vi "Set ROI HW lines limit.vi"(8 "error in (no error)":errorcluster) -> (0 "error out":errorcluster)   [LabVIEW 2020]
uses:
  Typedefs/HW config states enum.ctl
  Global Variables/General Globals.vi
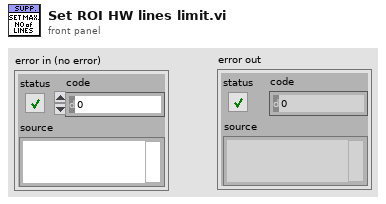
[diagram p1: front panel]
types:
  T1 = typedef "HW config states enum.ctl" = enum16{"Load from file", "Save to file", "Save backup", "Write all", "Read all", "Write XY stage settings", "Write DAQ FPGA settings", "Write Control FPGA settings", "Write Phys Channels", "Write System Config", "Write HW Config", "Save System Config", "Save HW Config", "Clear", "Compare from file"}
  T2 = typedef "Hardware Configuration settings.ctl" = cluster{"Dev. PC":bool, "Swap XY on stage":bool, "No of AOD":u8, "MC Supported":bool, "Axial MC":bool, "Computer MAC address":string, "Externalise Triggers":bool, "Trigger HW config":T3, "DAQmx Chan":T4, "XY stage available":bool, "XY Stage":T5, "Z stage available":bool, "Z Stage config cluster":T6, "Encoder available":bool, "Encoder":T7, "VidRec available":bool, "Cam VidRec":T8, "Laser Power Control HW config":T9, "Laser 1 available":bool, "Laser 1 config cluster":T10, "Prechirper 1 available":bool, "Prechirper 1 config cluster":T11, "Control system.FPGA available?":bool, "Control Sys. HW config":T12, "DAQ FPGA HW Config":T13, "PMT Voltage Range":T17}
  T3 = typedef "Triggers HW config.ctl" = cluster{"Available Device List":i32, "Device Address":string}
  T4 = typedef "DAQmx physical channels cluster.ctl" = cluster{"Pockels AO":tag, "Hard shutter AO":tag, "PMT AOs":tag, "Galvo AOs":tag, "Power meter AI":tag}
  T5 = typedef "XY Stage config cluster.ctl" = cluster{"COM port":refnum<visa-resource-name>, "Baudrate":i32, "Type":string}
  T6 = typedef "Z Stage config cluster.ctl" = cluster{"COM port":refnum<visa-resource-name>, "Baudrate":i32, "Type":string}
  T7 = typedef "Encoder config cluster.ctl" = cluster{"IP address":string, "Port":u16, "Wheel radius (cm)":dbl, "Encoder Trigger":tag}
  T8 = typedef "Cam VidRec HW config setup cluster.ctl" = cluster{"DO flag-Video record":tag, "DO flag-Trial start":tag}
  T9 = typedef "Laser Power Control HW config.ctl" = cluster{"Laser Power Control":string, "Laser Power Modulation Control":enum16{"NI", "FPGA"}}
  T10 = typedef "Laser 1 config cluster.ctl" = cluster{"COM port":refnum<visa-resource-name>, "Baud Rate":i32, "Type":string}
  T11 = typedef "PreChirper 1 config cluster.ctl" = cluster{"Type":string, "Baud Rate":i32, "COM port":refnum<visa-resource-name>}
  T12 = typedef "Control Sys HW config cluster.ctl" = cluster{"Control system.FPGA Type":enum16{"Virtex 5", "Virtex 7"}, "Control system.Network adapter name":string, "Control system.MAC address":string, "Control system.Ethernet Port":u32, "Control system.Ethernet Port Opened":bool}
  T13 = typedef "DAQ FPGA HW config cluster.ctl" = cluster{"FGPA Ref":T14, "Target":T15, "input card type":T16}
  T14 = typedef "FPGA Ref.ctl" = refnum<k20>
  T15 = typedef "nirio_resource_hc.ctl" = tag
  T16 = typedef "FPGA input type AC-DC.ctl" = enum16{"AC Card", "DC Card"}
  T17 = typedef "PMT Voltage Range.ctl" = cluster{"PMT Voltage Lower Limit":dbl, "PMT Voltage Upper Limit":dbl}
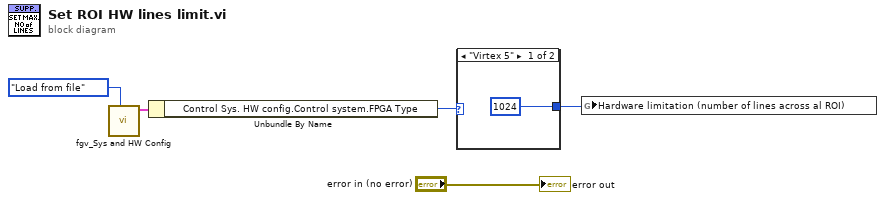
[diagram p0: block diagram]
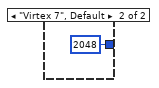
[diagram p2: hidden frame]
diagram:
  n1 = call "fgv_Sys and HW Config.vi"("Function"=HW_config_states_enum."Load from file") -> ("Hardware Configuration OUT"=w4:T2)  [unwired: 8 in, 2 out]
  n2 = Unbundle By Name(w4) -> ("Control Sys. HW config.Control system.FPGA Type"=w3:enum16{"Virtex 5", "Virtex 7"})
  n3 = case shown="\"Virtex 5\"" w3 {
    tunnel: [1024 ("Hardware limitation (number of lines across al ROI)") 2048 ("Hardware limitation (number of lines across al ROI)")] -> w2
    frame "Virtex 5" {
    }
    frame "Virtex 7", Default {
    }
  }
  n4 = global write "General Globals.vi" "Hardware limitation (number of lines across al ROI)"(w2) -> ()
  "error out" <- "error in (no error)"
